vi "Check P2.vi"(5 "Calibrated Results (P2 Left Edge Angles)":sgl[][](array[numeric]) format="%.2f", 7 "Calibrated Results (P2 Right Edge Angle)":sgl[][](array[numeric]) format="%.2f", 9 "P2 Hole":dbl, 11 "Error In":errorcluster) -> (1 "P2 Hole Status":bool, 2 "P2 Right Edge Angle Status":bool, 3 "P2 Left Edge Angle Status":bool, 6 "P2 Left Edge Angle":dbl, 8 "P2 Right Edge Angle":dbl, 10 "P2 Hole":dbl, 13 "P2 Status":bool caption="Status", 15 "Error Out":errorcluster)   [LabVIEW 2020]
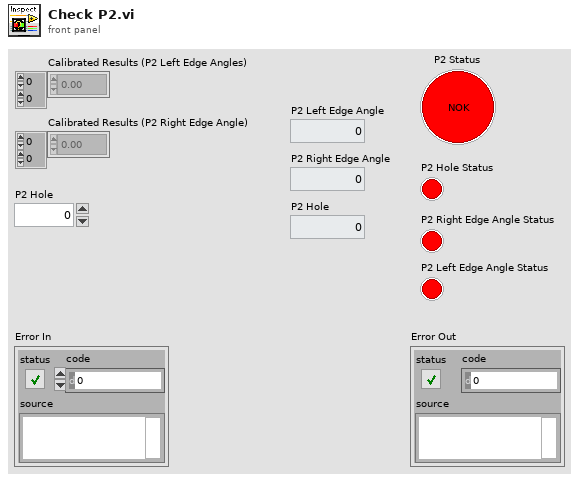
[diagram p1: front panel]
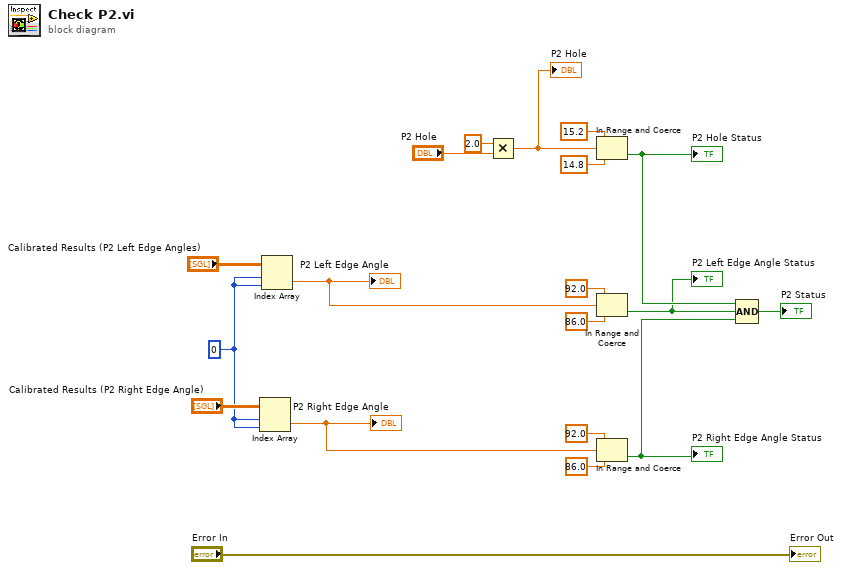
[diagram p0: block diagram]
diagram:
  w7 = 0 ("index (row)")
  n1 = Index Array(array="Calibrated Results (P2 Right Edge Angle)", index (row)=w7, index (col)=w7) -> (element=w5:sgl)
  "P2 Right Edge Angle" <- w5
  n2 = Index Array(array="Calibrated Results (P2 Left Edge Angles)", index (row)=w7, index (col)=w7) -> (element=w6:sgl)
  "P2 Left Edge Angle" <- w6
  n3 = Multiply(x=2.0, y="P2 Hole") -> (x*y=w1:dbl)
  "P2 Hole" <- w1
  n4 = In Range and Coerce(upper limit=15.2, x=w1, lower limit=14.8) -> (In Range?=w12:bool)  [unwired: 1 out]
  "P2 Hole Status" <- w12
  n5 = In Range and Coerce(upper limit=92.0, x=w6, lower limit=86.0) -> (In Range?=w11:bool)  [unwired: 1 out]
  "P2 Left Edge Angle Status" <- w11
  n6 = In Range and Coerce(upper limit=92.0, x=w5, lower limit=86.0) -> (In Range?=w10:bool)  [unwired: 1 out]
  "P2 Right Edge Angle Status" <- w10
  n7 = Compound Arithmetic op=AND(w12, w11, w10) -> (→"P2 Status":bool)
  "Error Out" <- "Error In"
